vi "Split.vi"(6 "Groups":string[][](array[string]), 8 "error in (no error)":errorcluster caption="entrée d'erreur (pas d'erreur)", 9 "y":string[][](array[string]), 10 "X":string[][](array[string]), 11 "RepeatedKFold.lvclass":refnum<class "RepeatedKFold.lvclass">) -> (0 "error out":errorcluster caption="sortie d'erreur", 2 "Split":T1(array[cluster]), 3 "RepeatedKFold.lvclass":refnum<class "RepeatedKFold.lvclass">)   [LabVIEW 2020, in "RepeatedKFold.lvclass"]
doc: "Returns : \n\n- train : ndarray\n The training set indices for that split.\n\n- test : ndarray\n The testing set indices for that split."
uses:
  RepeatedKFold.lvclass
  RepeatedKFold.lvclass/RepeatedKFold.ctl
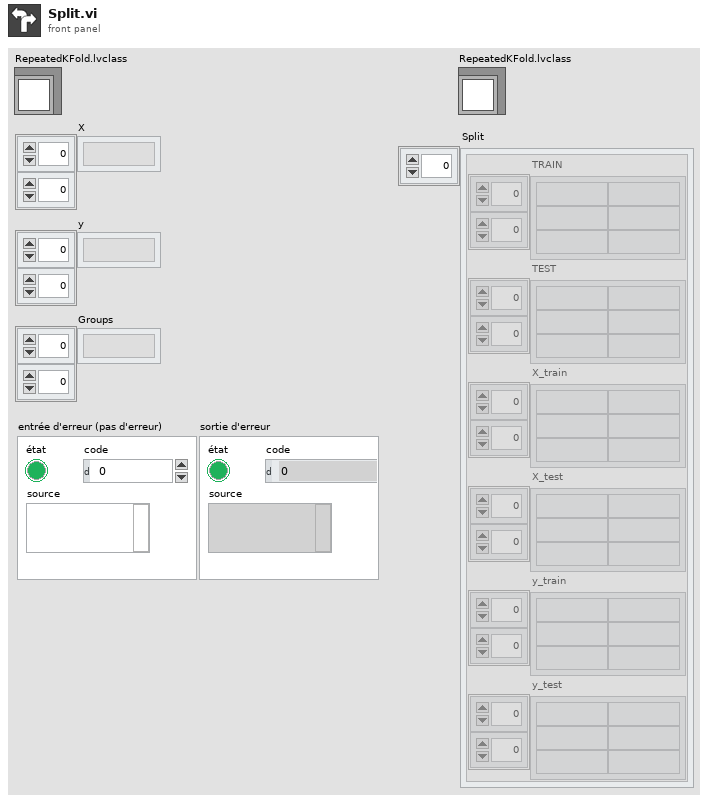
[diagram p1: front panel]
types:
  T1 = cluster{"TRAIN":string[][], "TEST":string[][], "X_train":string[][], "X_test":string[][], "y_train":string[][], "y_test":string[][]}[]
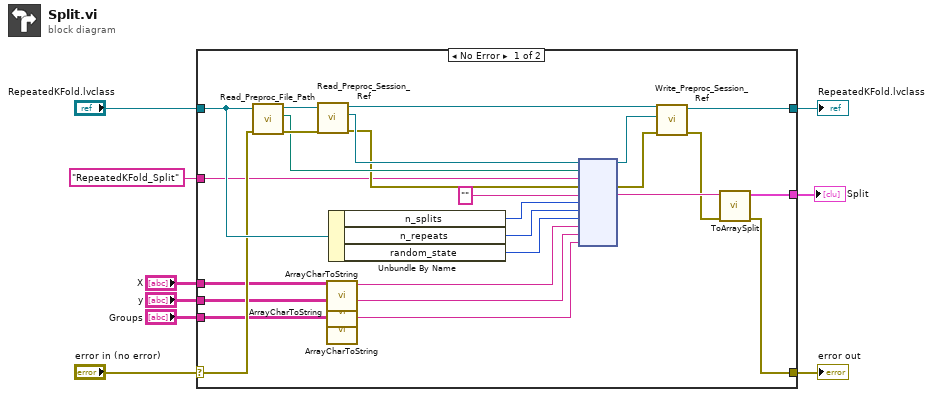
[diagram p0: block diagram]
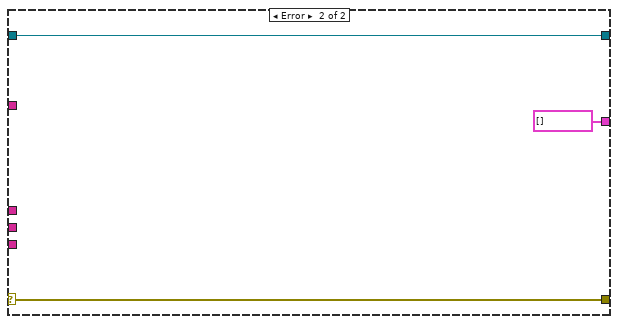
[diagram p2: hidden frame]
diagram:
  n1 = case shown="No Error" "error in (no error)" {
    selector: "error in (no error)" -> [w25 w38]
    tunnel: [w11 w38] -> w8
    tunnel: [w17 w37] -> w6
    tunnel: "RepeatedKFold.lvclass" -> [w26 w37]
    tunnel: "RepeatedKFold_Split" -> [w24 _]
    tunnel: "X" -> [w16 _]
    tunnel: "y" -> [w15 _]
    tunnel: "Groups" -> [w14 _]
    tunnel: [w10 T1 [] ("Split")] -> w1
    frame No Error {
      n2 = call-dynamic "Read_Preproc_File_Path.vi"("error in (no error)"=w25, "Python in"=w26) -> ("error out"=w34:errorcluster, "File_Path"=w33:path, "Python out"=w35:refnum<class "RepeatedKFold.lvclass">)  [unwired: 7 in]
      n3 = call-dynamic "Read_Preproc_Session_Ref.vi"("error in (no error)"=w34, "Python in"=w35) -> ("error out"=w31:errorcluster, "Session_ref"=w32:refnum<k35>, "Python out"=w30:refnum<class "RepeatedKFold.lvclass">)  [unwired: 7 in]
      n4 = call "ArrayCharToString.vi"("TAB"=w16) -> ("Instruction"=w20:string)  [unwired: 10 in]
      n5 = call "ArrayCharToString.vi"("TAB"=w15) -> ("Instruction"=w19:string)  [unwired: 10 in]
      n6 = call "ArrayCharToString.vi"("TAB"=w14) -> ("Instruction"=w18:string)  [unwired: 10 in]
      n7 = Unbundle By Name(w26) -> ("n_splits"=w23:i32, "n_repeats"=w22:i32, "random_state"=w21:i32)
      n8 = node(w32, w33, w24, w31, "", w23, w22, w21, w20, w19, w18) -> (w28:refnum<k35>, w29:errorcluster, w13:string)  [unwired: 6 in, 2 out]
      n9 = call-dynamic "Write_Preproc_Session_Ref.vi"("error in (no error)"=w29, "Session_ref"=w28, "Python in"=w30) -> ("error out"=w12:errorcluster, "Python out"=w17:refnum<class "RepeatedKFold.lvclass">)  [unwired: 7 in]
      n10 = call "ToArraySplit.vi"("sortie d'erreur"=w12, "Return value"=w13) -> ("sortie d'erreur"=w11:errorcluster, "Split"=w10:T1)  [unwired: 8 in]
    }
    frame Error {
    }
  }
  "error out" <- w8
  "RepeatedKFold.lvclass" <- w6
  "Split" <- w1
